vi "Global Data FGV.vi"(10 "Global Data In":T2, 11 "Operation":T1(ring)) -> (2 "Global Data Out":T2)   [LabVIEW 2010]
uses:
  Global Data.ctl
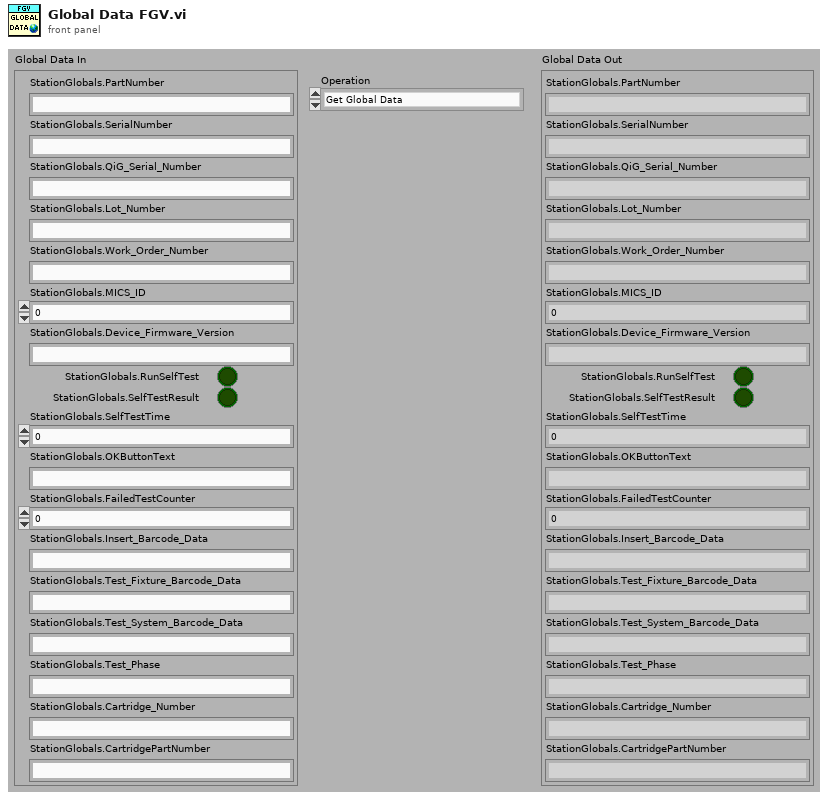
[diagram p1: front panel]
types:
  T1 = enum16{"Get Global Data", "Set Global Data", "Reset Global Data"}
  T2 = typedef "Global Data.ctl" = cluster{"StationGlobals.PartNumber":string, "StationGlobals.SerialNumber":string, "StationGlobals.QiG_Serial_Number":string, "StationGlobals.Lot_Number":string, "StationGlobals.Work_Order_Number":string, "StationGlobals.MICS_ID":dbl, "StationGlobals.Device_Firmware_Version":string, "StationGlobals.OKButtonText":string, "StationGlobals.Insert_Barcode_Data":string, "StationGlobals.RunSelfTest":bool, "StationGlobals.SelfTestResult":bool, "StationGlobals.SelfTestTime":dbl, "StationGlobals.FailedTestCounter":dbl, "StationGlobals.Test_Fixture_Barcode_Data":string, "StationGlobals.Test_System_Barcode_Data":string, "StationGlobals.Test_Phase":string, "StationGlobals.Cartridge_Number":string, "StationGlobals.CartridgePartNumber":string}
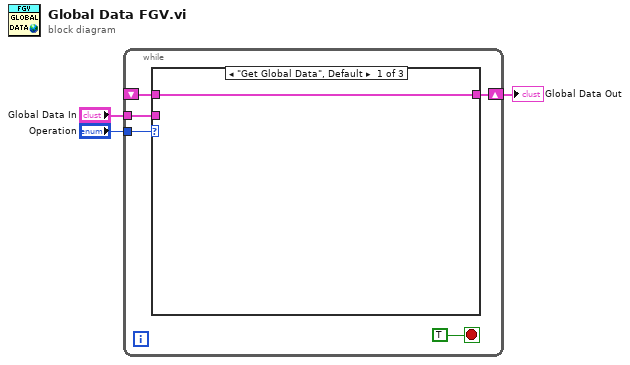
[diagram p0: block diagram]
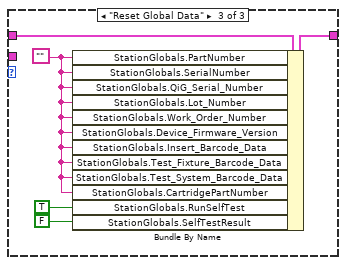
[diagram p3: hidden frame]
diagram:
  n1 = while {
    shift-right: [w6] -> w1
    shift-left: _ -> [w5]
    tunnel: "Operation" -> [w8]
    tunnel: "Global Data In" -> [w7]
    stop <- TRUE stop-if-true
    n2 = case shown="\"Get Global Data\", Default" w8 {
      tunnel: w7 -> [_ w10 _]
      tunnel: [w9 w10 w14] -> w6
      tunnel: w5 -> [w9 _ w15]
      frame "Get Global Data", Default {
      }
      frame "Set Global Data" {
      }
      frame "Reset Global Data" {
        w11 = ""
        n3 = Bundle By Name(cluster=w15, "StationGlobals.PartNumber"=w11, "StationGlobals.SerialNumber"=w11, "StationGlobals.QiG_Serial_Number"=w11, "StationGlobals.Lot_Number"=w11, "StationGlobals.Work_Order_Number"=w11, "StationGlobals.Device_Firmware_Version"=w11, "StationGlobals.Insert_Barcode_Data"=w11, "StationGlobals.Test_Fixture_Barcode_Data"=w11, "StationGlobals.Test_System_Barcode_Data"=w11, "StationGlobals.CartridgePartNumber"=w11, "StationGlobals.RunSelfTest"=TRUE, "StationGlobals.SelfTestResult"=FALSE) -> (w14:T2)
      }
    }
  }
  "Global Data Out" <- w1
